vi "initialize.vi"(8 "error in (no error)":errorcluster, 11 "Experiment in":refnum<class "Experiment.lvclass">) -> (0 "error out":errorcluster, 3 "Experiment out":refnum<class "Experiment.lvclass">)   [LabVIEW 2014, in "Experiment.lvclass"]
uses:
  Experiment.lvclass
  Experiment.lvclass/Experiment.ctl
  Globals.vi
  Camera/Hamamatsu_C9100-13/Hamamatsu_C9100-13.lvclass
  HSDIO/HSDIO.lvclass
  Counter/Counter.lvclass
  PI_piezo/PI_Piezo.lvclass
  TTL_input/TTL_input.lvclass
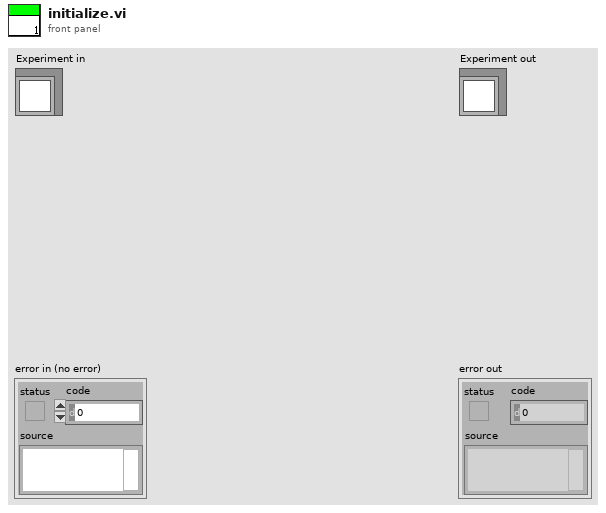
[diagram p1: front panel]
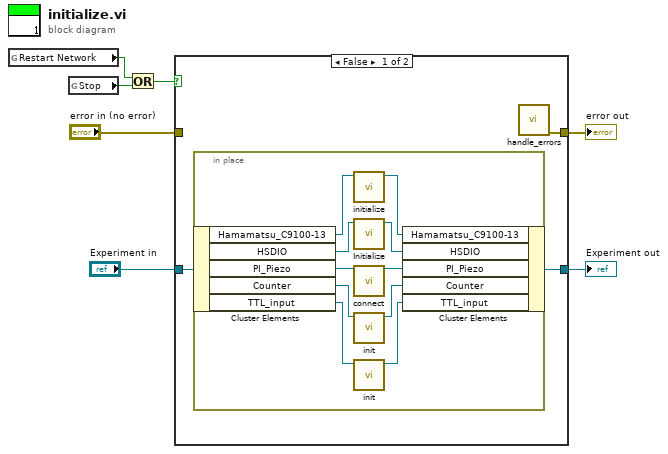
[diagram p0: block diagram]
diagram:
  n1 = global read "Globals.vi" "Restart Network"() -> (w4:bool)
  n2 = global read "Globals.vi" "Stop"() -> (w3:bool)
  n3 = Or(x=w4, y=w3) -> (x .or. y?=w2:bool)
  n4 = case shown="False" w2 {
    tunnel: [w8 w21] -> w7
    tunnel: [w9 w22] -> w5
    tunnel: "Experiment in" -> [w10 w22]
    tunnel: "error in (no error)" -> [_ w21]
    frame False {
      n5 = in-place {
        n6 = in-place-cluster #1(w10) -> ("Hamamatsu_C9100-13"=w20:refnum<class "Hamamatsu_C9100-13.lvclass">, "HSDIO"=w17:refnum<class "HSDIO.lvclass">, "PI_Piezo"=w16:refnum<class "PI_Piezo.lvclass">, "Counter"=w11:refnum<class "Counter.lvclass">, "TTL_input"=w12:refnum<class "TTL_input.lvclass">)
        n7 = call-dynamic "initialize.vi"("Hamamatsu_C9100-13 in"=w20) -> ("Hamamatsu_C9100-13 out"=w19:refnum<class "Hamamatsu_C9100-13.lvclass">)  [unwired: 9 in, 1 out]
        n8 = call "Initialize.vi"("HSDIO in"=w17) -> ("HSDIO out"=w18:refnum<class "HSDIO.lvclass">)  [unwired: 9 in, 1 out]
        n9 = call "connect.vi"("PI_Piezo.lvclass (in)"=w16) -> ("PI_Piezo.lvclass"=w15:refnum<class "PI_Piezo.lvclass">)  [unwired: 13 in, 1 out]
        n10 = call "init.vi"("Counter in"=w11) -> ("Counter out"=w14:refnum<class "Counter.lvclass">)  [unwired: 9 in, 1 out]
        n11 = call "init.vi"("TTL_input.lvclass"=w12) -> ("TTL_input out"=w13:refnum<class "TTL_input.lvclass">)  [unwired: 9 in, 1 out]
        n12 = in-place-cluster #1("Hamamatsu_C9100-13"=w19, "HSDIO"=w18, "PI_Piezo"=w15, "Counter"=w14, "TTL_input"=w13) -> (w9:refnum<class "Experiment.lvclass">)
      }
      n13 = call "handle_errors.vi"() -> ("error out"=w8:errorcluster)  [unwired: 15 in]
    }
    frame True {
    }
  }
  "error out" <- w7
  "Experiment out" <- w5
